vi "AB_RW_Project_EXE_ActiveX_Info.vi"(7 "action":T1, 8 "error in (no error)":errorcluster, 10 "activeX info in":T2, 11 "Object In":T3) -> (0 "error out":errorcluster, 2 "activeX info out":T2, 3 "Object Out":T3, 5 "empty":bool)   [LabVIEW 2020]
uses:
  <resource>/Framework/Providers/API/ItemRef.ctl
  <vilib>/AppBuilder/RW_Project/AB_RW_Project_EXE_ActiveX_Data.ctl
  <vilib>/AppBuilder/RW_Project/AB_RW_Project_PropBag_Action.ctl
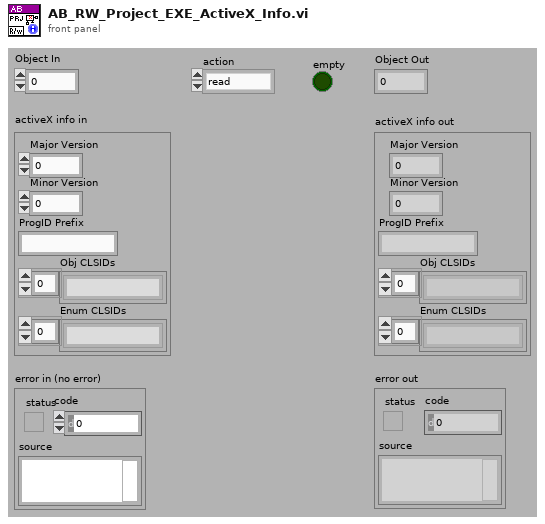
[diagram p1: front panel]
types:
  T1 = typedef "AB_RW_Project_PropBag_Action.ctl" = enum16{"read", "write", "clear", "readPrevious", "writePrevious", "clearPrevious"}
  T2 = typedef "AB_RW_Project_EXE_ActiveX_Data.ctl" = cluster{"Major Version":u16, "Minor Version":u16, "ProgID Prefix":string, "Obj CLSIDs":string[], "Enum CLSIDs":string[]}
  T3 = typedef "ItemRef.ctl" = u64
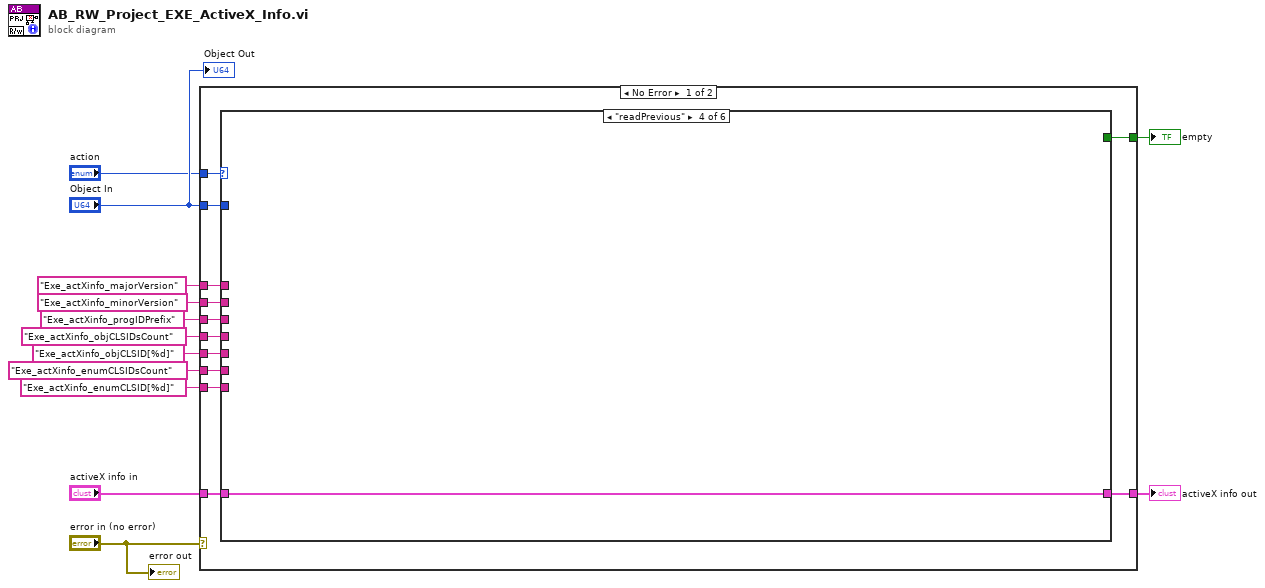
[diagram p0: block diagram]
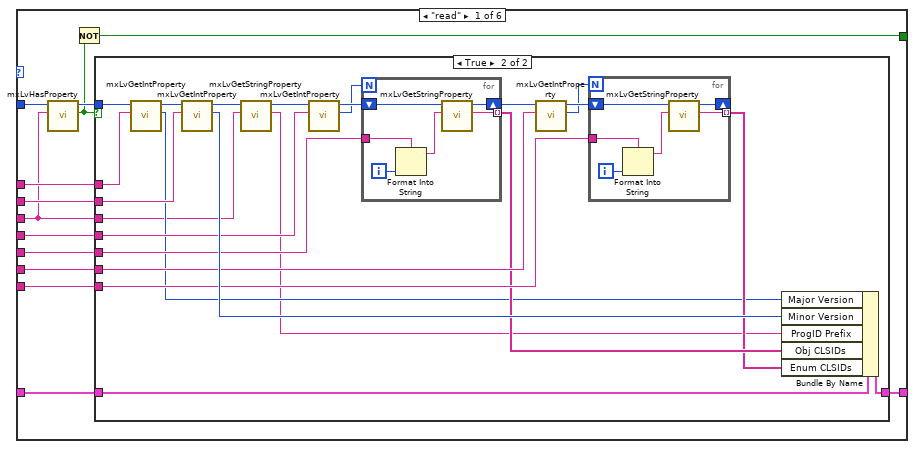
[diagram p2: hidden frame]
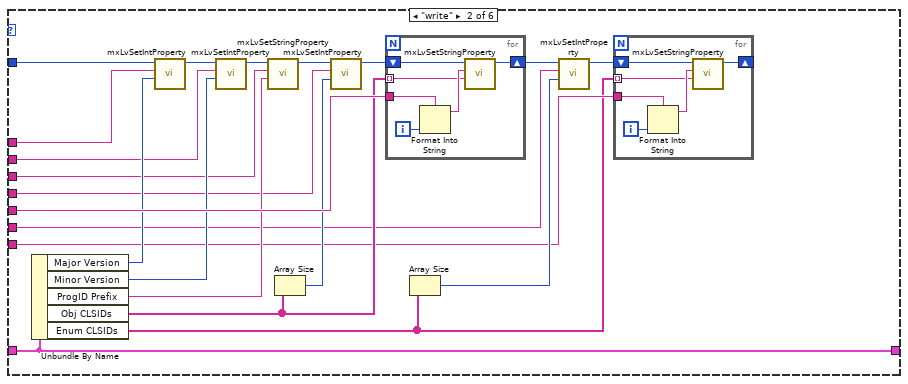
[diagram p4: hidden frame]
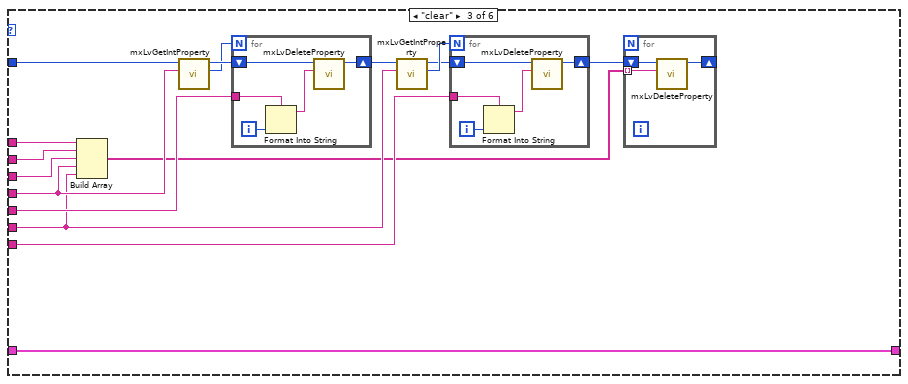
[diagram p5: hidden frame]
diagram:
  n1 = case shown="No Error" "error in (no error)" {
    tunnel: "Object In" -> [w23 _]
    tunnel: [w25 _] -> w11
    tunnel: "Exe_actXinfo_majorVersion" -> [w24 _]
    tunnel: "Exe_actXinfo_minorVersion" -> [w22 _]
    tunnel: "Exe_actXinfo_progIDPrefix" -> [w21 _]
    tunnel: "activeX info in" -> [w20 _]
    tunnel: "action" -> [w19 _]
    tunnel: "Exe_actXinfo_objCLSIDsCount" -> [w18 _]
    tunnel: "Exe_actXinfo_objCLSID[%d]" -> [w17 _]
    tunnel: "Exe_actXinfo_enumCLSIDsCount" -> [w16 _]
    tunnel: "Exe_actXinfo_enumCLSID[%d]" -> [w15 _]
    tunnel: [w14 _] -> w1
    frame No Error {
      n2 = case shown="\"readPrevious\"" w19 {
        tunnel: [w38 w93 w124 w138 w139 w140] -> w25
        tunnel: w24 -> [w36 w94 w123 _ _ _]
        tunnel: w23 -> [w30 w95 w118 _ _ _]
        tunnel: w22 -> [w35 w90 w122 _ _ _]
        tunnel: w21 -> [w28 w87 w121 _ _ _]
        tunnel: w20 -> [w37 w93 w124 w138 w139 w140]
        tunnel: w18 -> [w34 w84 w117 _ _ _]
        tunnel: w17 -> [w33 w96 w116 _ _ _]
        tunnel: w16 -> [w32 w77 w112 _ _ _]
        tunnel: w15 -> [w31 w76 w111 _ _ _]
        tunnel: [w26 _ _ _ _ _] -> w14
        frame "read" {
          n3 = call <resource>:"mxLvHasProperty.vi"("Tag"=w28, "Item"=w30) -> ("HasProperty"=w27:bool, "Item"=w29:T3)  [unwired: 7 in, 1 out]
          n4 = Not(x=w27) -> (.not. x?=w26:bool)
          n5 = case shown="True" w27 {
            tunnel: [w39 w62] -> w38
            tunnel: w37 -> [w39 w61]
            tunnel: w36 -> [_ w59]
            tunnel: w35 -> [_ w58]
            tunnel: w34 -> [_ w55]
            tunnel: w33 -> [_ w53]
            tunnel: w32 -> [_ w49]
            tunnel: w31 -> [_ w48]
            tunnel: w29 -> [_ w43]
            tunnel: w28 -> [_ w42]
            frame False {
            }
            frame True {
              n6 = call <resource>:"mxLvGetIntProperty.vi"("Tag"=w59, "Item"=w43) -> ("Value"=w45:i32, "Item"=w60:T3)  [unwired: 7 in, 1 out]
              n7 = call <resource>:"mxLvGetIntProperty.vi"("Tag"=w58, "Item"=w60) -> ("Value"=w56:i32, "Item"=w57:T3)  [unwired: 7 in, 1 out]
              n8 = call <resource>:"mxLvGetStringProperty.vi"("Tag"=w42, "Item"=w57) -> ("Value"=w44:string, "Item"=w54:T3)  [unwired: 7 in, 1 out]
              n9 = call <resource>:"mxLvGetIntProperty.vi"("Tag"=w55, "Item"=w54) -> ("Value"=w41:i32, "Item"=w52:T3)  [unwired: 7 in, 1 out]
              n10 = for {
                N: w41 -> [_]
                tunnel: w53 -> [w74]
                shift-right: [w71] -> w50
                shift-left: w52 -> [w72]
                tunnel: [w69] -> w47 mode=indexing
                i -> [w73]
                n11 = Format Into String(format string=w74, w73) -> (resulting string=w70:string)  [unwired: 2 in, 1 out]
                n12 = call <resource>:"mxLvGetStringProperty.vi"("Tag"=w70, "Item"=w72) -> ("Value"=w69:string, "Item"=w71:T3)  [unwired: 7 in, 1 out]
              }
              n13 = call <resource>:"mxLvGetIntProperty.vi"("Tag"=w49, "Item"=w50) -> ("Value"=w40:i32, "Item"=w51:T3)  [unwired: 7 in, 1 out]
              n14 = for {
                N: w40 -> [_]
                tunnel: w48 -> [w68]
                shift-right: [w65] -> _
                shift-left: w51 -> [w66]
                tunnel: [w63] -> w46 mode=indexing
                i -> [w67]
                n15 = Format Into String(format string=w68, w67) -> (resulting string=w64:string)  [unwired: 2 in, 1 out]
                n16 = call <resource>:"mxLvGetStringProperty.vi"("Tag"=w64, "Item"=w66) -> ("Value"=w63:string, "Item"=w65:T3)  [unwired: 7 in, 1 out]
              }
              n17 = Bundle By Name(cluster=w61, "Major Version"=w45, "Minor Version"=w56, "ProgID Prefix"=w44, "Obj CLSIDs"=w47, "Enum CLSIDs"=w46) -> (w62:T2)
            }
          }
        }
        frame "write" {
          n18 = Unbundle By Name(w93) -> ("Major Version"=w92:u16, "Minor Version"=w89:u16, "ProgID Prefix"=w86:string, "Obj CLSIDs"=w81:string[], "Enum CLSIDs"=w75:string[])
          n19 = call <resource>:"mxLvSetIntProperty.vi"("Value (0)"=w92, "Tag"=w94, "Item"=w95) -> ("Item"=w91:T3)  [unwired: 7 in, 1 out]
          n20 = call <resource>:"mxLvSetIntProperty.vi"("Value (0)"=w89, "Tag"=w90, "Item"=w91) -> ("Item"=w88:T3)  [unwired: 7 in, 1 out]
          n21 = call <resource>:"mxLvSetStringProperty.vi"("Value (\"\")"=w86, "Tag"=w87, "Item"=w88) -> ("Item"=w85:T3)  [unwired: 7 in, 1 out]
          n22 = Array Size(array=w81) -> (size(s)=w82:i32)
          n23 = call <resource>:"mxLvSetIntProperty.vi"("Value (0)"=w82, "Tag"=w84, "Item"=w85) -> ("Item"=w83:T3)  [unwired: 7 in, 1 out]
          n24 = for {
            tunnel: w96 -> [w108]
            shift-right: [w105] -> w79
            shift-left: w83 -> [w106]
            tunnel: w81 -> [w103] mode=indexing
            i -> [w107]
            n25 = Format Into String(format string=w108, w107) -> (resulting string=w104:string)  [unwired: 2 in, 1 out]
            n26 = call <resource>:"mxLvSetStringProperty.vi"("Value (\"\")"=w103, "Tag"=w104, "Item"=w106) -> ("Item"=w105:T3)  [unwired: 7 in, 1 out]
          }
          n27 = Array Size(array=w75) -> (size(s)=w78:i32)
          n28 = call <resource>:"mxLvSetIntProperty.vi"("Value (0)"=w78, "Tag"=w77, "Item"=w79) -> ("Item"=w80:T3)  [unwired: 7 in, 1 out]
          n29 = for {
            tunnel: w76 -> [w102]
            shift-right: [w99] -> _
            shift-left: w80 -> [w100]
            tunnel: w75 -> [w97] mode=indexing
            i -> [w101]
            n30 = Format Into String(format string=w102, w101) -> (resulting string=w98:string)  [unwired: 2 in, 1 out]
            n31 = call <resource>:"mxLvSetStringProperty.vi"("Value (\"\")"=w97, "Tag"=w98, "Item"=w100) -> ("Item"=w99:T3)  [unwired: 7 in, 1 out]
          }
        }
        frame "clear" {
          n32 = Build Array(w123, w122, w121, w117, w112) -> (w110:string[])
          n33 = call <resource>:"mxLvGetIntProperty.vi"("Tag"=w117, "Item"=w118) -> ("Value"=w119:i32, "Item"=w120:T3)  [unwired: 7 in, 1 out]
          n34 = for {
            N: w119 -> [_]
            tunnel: w116 -> [w137]
            shift-right: [w134] -> w113
            shift-left: w120 -> [w135]
            i -> [w136]
            n35 = Format Into String(format string=w137, w136) -> (resulting string=w133:string)  [unwired: 2 in, 1 out]
            n36 = call <resource>:"mxLvDeleteProperty.vi"("Tag"=w133, "Item"=w135) -> ("Item"=w134:T3)  [unwired: 8 in, 1 out]
          }
          n37 = call <resource>:"mxLvGetIntProperty.vi"("Tag"=w112, "Item"=w113) -> ("Value"=w115:i32, "Item"=w114:T3)  [unwired: 7 in, 1 out]
          n38 = for {
            N: w115 -> [_]
            tunnel: w111 -> [w132]
            shift-right: [w129] -> w109
            shift-left: w114 -> [w130]
            i -> [w131]
            n39 = Format Into String(format string=w132, w131) -> (resulting string=w128:string)  [unwired: 2 in, 1 out]
            n40 = call <resource>:"mxLvDeleteProperty.vi"("Tag"=w128, "Item"=w130) -> ("Item"=w129:T3)  [unwired: 8 in, 1 out]
          }
          n41 = for {
            shift-right: [w126] -> _
            shift-left: w109 -> [w127]
            tunnel: w110 -> [w125] mode=indexing
            n42 = call <resource>:"mxLvDeleteProperty.vi"("Tag"=w125, "Item"=w127) -> ("Item"=w126:T3)  [unwired: 8 in, 1 out]
          }
        }
        frame "readPrevious" {
        }
        frame "writePrevious" {
        }
        frame "clearPrevious" {
        }
      }
    }
    frame Error {
    }
  }
  "activeX info out" <- w11
  "empty" <- w1
  "Object Out" <- "Object In"
  "error out" <- "error in (no error)"
